vi "Write Local Resource.vi"(8 "error in (no error)":errorcluster, 10 "Local Resource":refnum<visa-resource-name>, 11 "SimELoad in":refnum<class "SimEload.lvclass">) -> (0 "error out":errorcluster, 3 "SimELoad out":refnum<class "SimEload.lvclass">)   [LabVIEW 2019, in "SimELoad.lvlib" / "SimEload.lvclass"]
uses:
  SimEload.lvclass
  SimEload.lvclass/SimEload.ctl
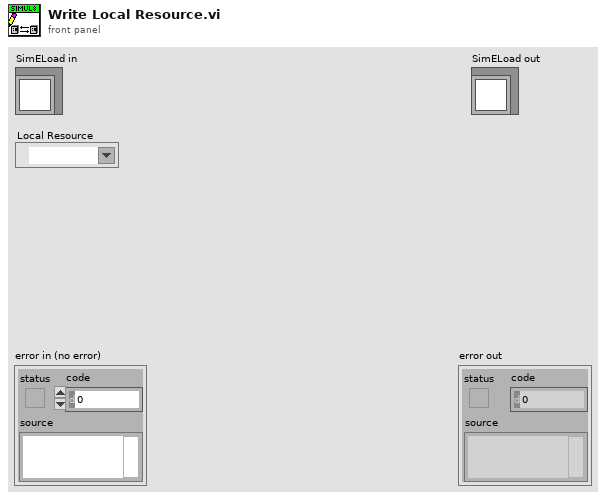
[diagram p1: front panel]
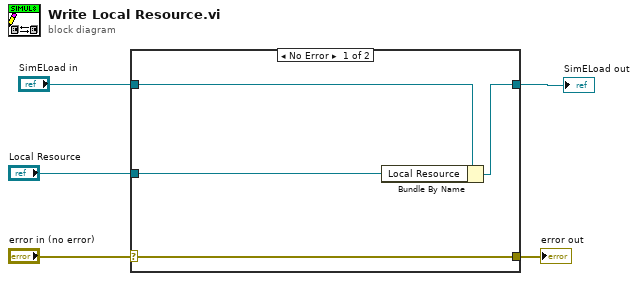
[diagram p0: block diagram]
diagram:
  n1 = case shown="No Error" "error in (no error)" {
    selector: "error in (no error)" -> [w9 w10]
    tunnel: [w9 w10] -> w4
    tunnel: [w7 w11] -> w1
    tunnel: "SimELoad in" -> [w8 w11]
    tunnel: "Local Resource" -> [w6 _]
    frame No Error {
      n2 = Bundle By Name(cluster=w8, "Local Resource"=w6) -> (w7:refnum<class "SimEload.lvclass">)
    }
    frame Error {
    }
  }
  "error out" <- w4
  "SimELoad out" <- w1
